vi "myPID.vi"(4 "s":bool, 7 "output range":cluster{"output high":dbl, "output low":dbl}={"output high"=100.0, "output low"=-100.0} {"output low" format="%.2f"; "output high" format="%.2f"}, 8 "Processer":dbl, 9 "setpoint":dbl, 11 "PID":cluster{"Kp":dbl, "Ki":dbl, "Kd":dbl}) -> (1 "out":dbl, 6 "e(t)":dbl)   [LabVIEW 2019]
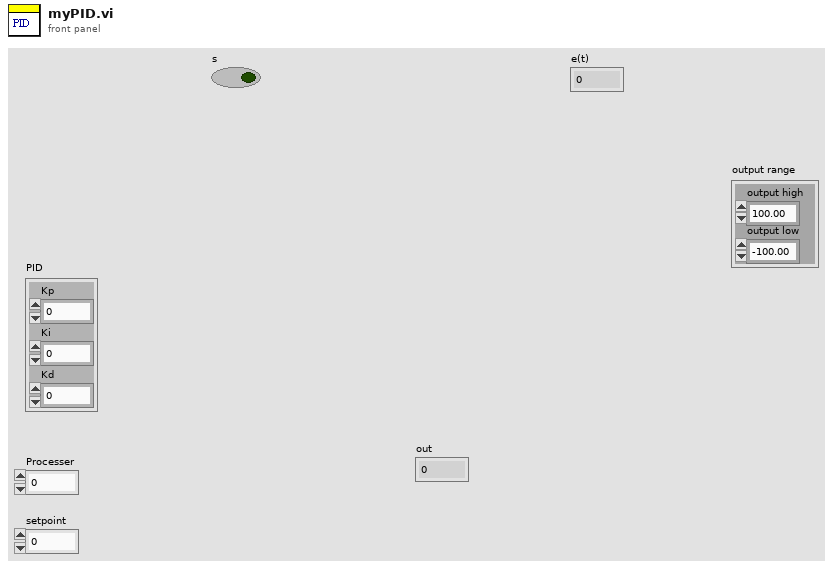
[diagram p1: front panel]
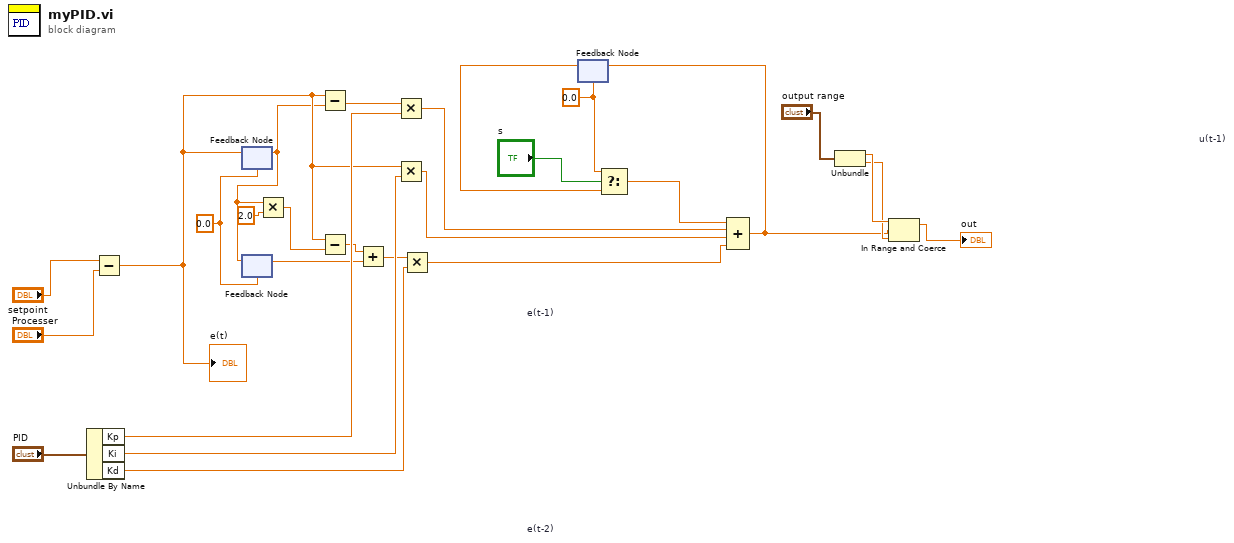
[diagram p0: block diagram]
diagram:
  w24 = 0.0
  w2 = 0.0
  n1 = Unbundle By Name("PID") -> ("Kp"=w22:dbl, "Ki"=w21:dbl, "Kd"=w13:dbl)
  n2 = Subtract(x="setpoint", y="Processer") -> (x-y=w20:dbl)
  "e(t)" <- w20
  n3 = feedback-in #1(w20) -> ()
  n4 = feedback #1 "e(t-1)"(w24) -> (w19:dbl)
  n5 = feedback #2 "e(t-2)"(w24) -> (w15:dbl)
  n6 = feedback-in #2(w19) -> ()
  n7 = Multiply(x=w19, y=2.0) -> (x*y=w17:dbl)
  n8 = Subtract(x=w20, y=w19) -> (x-y=w23:dbl)
  n9 = Subtract(x=w20, y=w17) -> (x-y=w16:dbl)
  n10 = Add(x=w16, y=w15) -> (x+y=w14:dbl)
  n11 = Multiply(x=w23, y=w22) -> (x*y=w10:dbl)
  n12 = Multiply(x=w20, y=w21) -> (x*y=w11:dbl)
  n13 = Multiply(x=w14, y=w13) -> (x*y=w12:dbl)
  n14 = feedback #3 "u(t-1)"(w2) -> (w3:dbl)
  n15 = Select(t=w2, s="s", f=w3) -> (s? t:f=w4:dbl)
  n16 = Compound Arithmetic op=ADD(w4, w10, w11, w12) -> (w6:dbl)
  n17 = feedback-in #3(w6) -> ()
  n18 = Unbundle("output range") -> ("output high"=w9:dbl, "output low"=w8:dbl)
  n19 = In Range and Coerce(upper limit=w9, x=w6, lower limit=w8) -> (coerced(x)=→"out":dbl)  [unwired: 1 out]
